vi "Festo Display.vi"() -> ()   [LabVIEW 2011]
uses:
  GlobalVariables.vi
panel:
  in  "Read/Write":bool
  in  "Festo Block 8":bool[][](array[boolean])=[[FALSE, FALSE], [FALSE, FALSE], [FALSE, FALSE], [FALSE, FALSE], [FALSE, FALSE], [FALSE, FALSE], [FALSE, FALSE], [FALSE, FALSE]]
  in  "Festo Block 7":bool[][](array[boolean])=[[FALSE, FALSE], [FALSE, FALSE], [FALSE, FALSE], [FALSE, FALSE], [FALSE, FALSE], [FALSE, FALSE], [FALSE, FALSE], [FALSE, FALSE]]
  in  "Festo Block 6":bool[][](array[boolean])=[[FALSE, FALSE], [FALSE, FALSE], [FALSE, FALSE], [FALSE, FALSE], [FALSE, FALSE], [FALSE, FALSE], [FALSE, FALSE], [FALSE, FALSE]]
  in  "Festo Block 5":bool[][](array[boolean])=[[FALSE, FALSE], [FALSE, FALSE], [FALSE, FALSE], [FALSE, FALSE], [FALSE, FALSE], [FALSE, FALSE], [FALSE, FALSE], [FALSE, FALSE]]
  in  "Festo Block 4":bool[][](array[boolean])=[[FALSE, FALSE], [FALSE, FALSE], [FALSE, FALSE], [FALSE, FALSE], [FALSE, FALSE], [FALSE, FALSE], [FALSE, FALSE], [FALSE, FALSE]]
  in  "Festo Block 3":bool[][](array[boolean])=[[FALSE, FALSE], [FALSE, FALSE], [FALSE, FALSE], [FALSE, FALSE], [FALSE, FALSE], [FALSE, FALSE], [FALSE, FALSE], [FALSE, FALSE]]
  in  "Festo Block 2":bool[][](array[boolean])=[[FALSE, FALSE], [FALSE, FALSE], [FALSE, FALSE], [FALSE, FALSE], [FALSE, FALSE], [FALSE, FALSE], [FALSE, FALSE], [FALSE, FALSE]]
  in  "Festo Block 1":bool[][](array[boolean])=[[FALSE, FALSE], [FALSE, FALSE], [FALSE, FALSE], [FALSE, FALSE], [FALSE, FALSE], [FALSE, FALSE], [FALSE, FALSE], [FALSE, FALSE]]
  in  "Close All Valves":bool
  in  "stop":bool
  # "79\n77\n75\n73\n71\n69\n67\n65"
  # "80\n78\n76\n74\n72\n70\n68\n66"
  # "50\n52\n54\n56\n58\n60\n62\n64"
  # "49\n51\n53\n55\n57\n59\n61\n63"
  # "95\n93\n91\n89\n87\n85\n83\n81"
  # "96\n94\n92\n90\n88\n86\n84\n82"
  # "34\n36\n38\n40\n42\n44\n46\n48"
  # "33\n35\n37\n39\n41\n43\n45\n47"
  # "111\n109\n107\n105\n103\n101\n99\n97"
  # "112\n110\n108\n106\n104\n102\n100\n98"
  # "18\n20\n22\n24\n26\n28\n30\n32"
  # "17\n19\n21\n23\n25\n27\n29\n31"
  # "127\n125\n123\n121\n119\n117\n115\n113"
  # "128\n126\n124\n122\n120\n118\n116\n114"
  # "2\n4\n6\n8\n10\n12\n14\n16"
  # "1\n3\n5\n7\n9\n11\n13\n15"
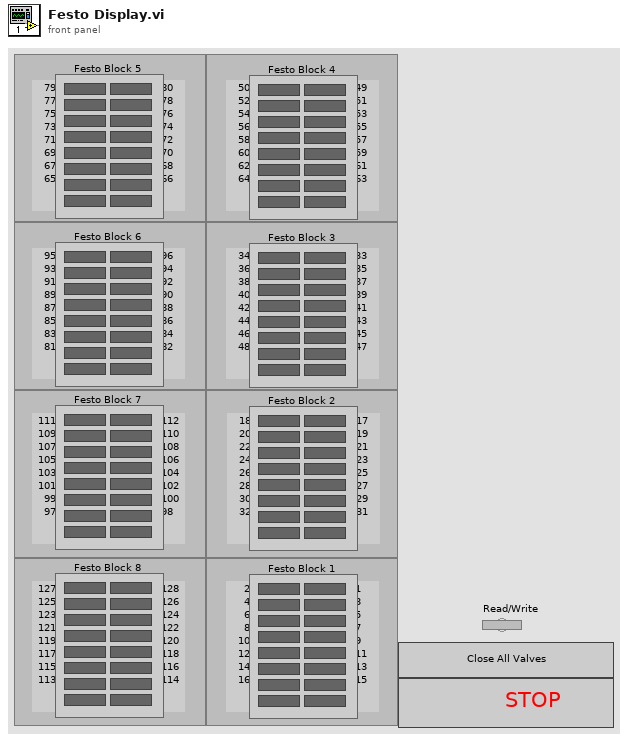
[diagram p1: front panel]
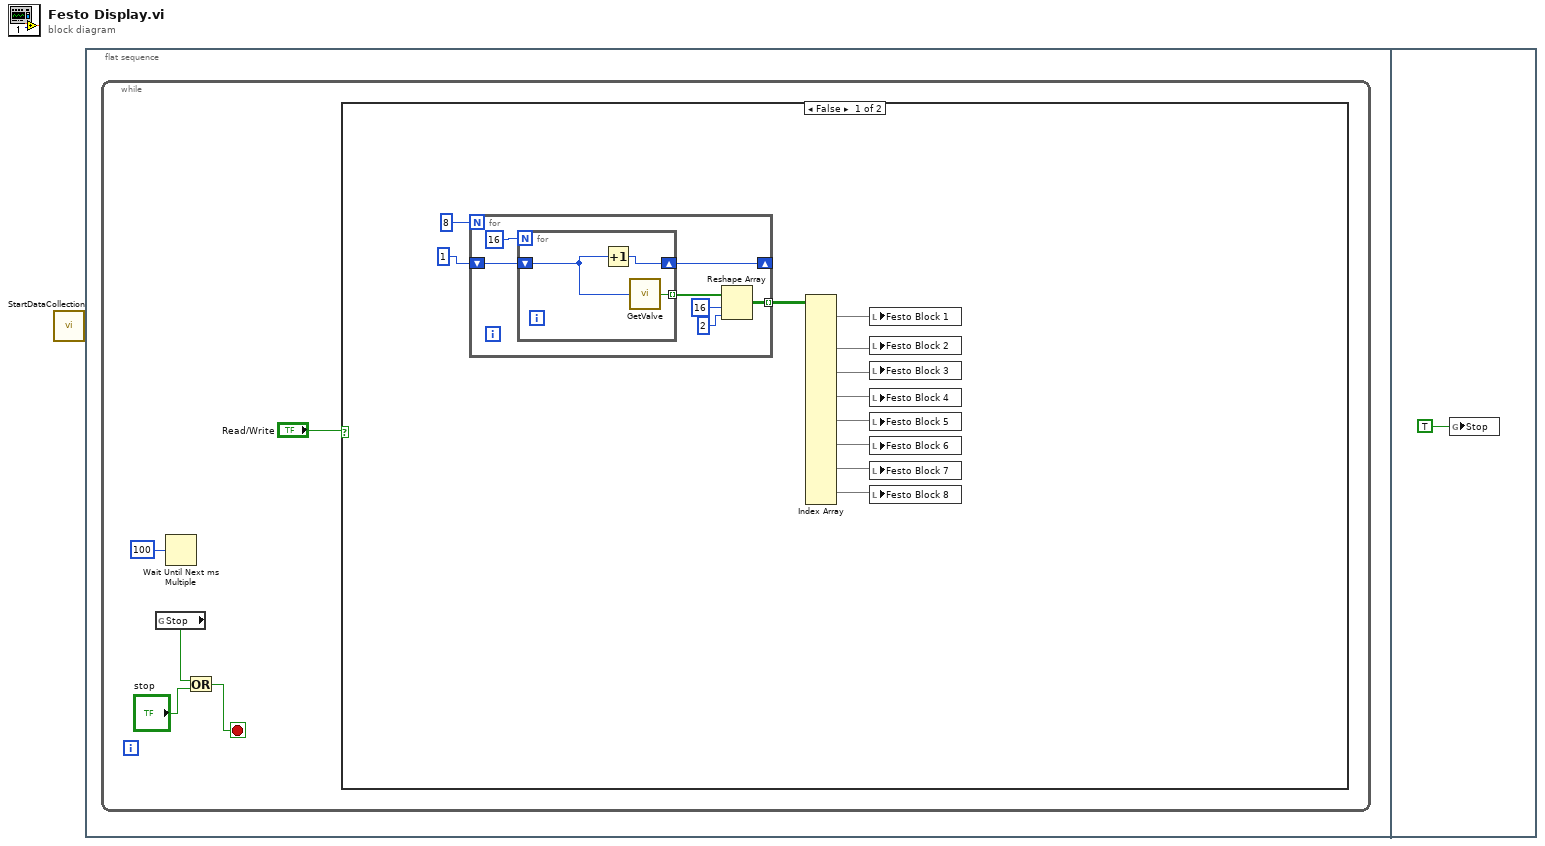
[diagram p0: block diagram]
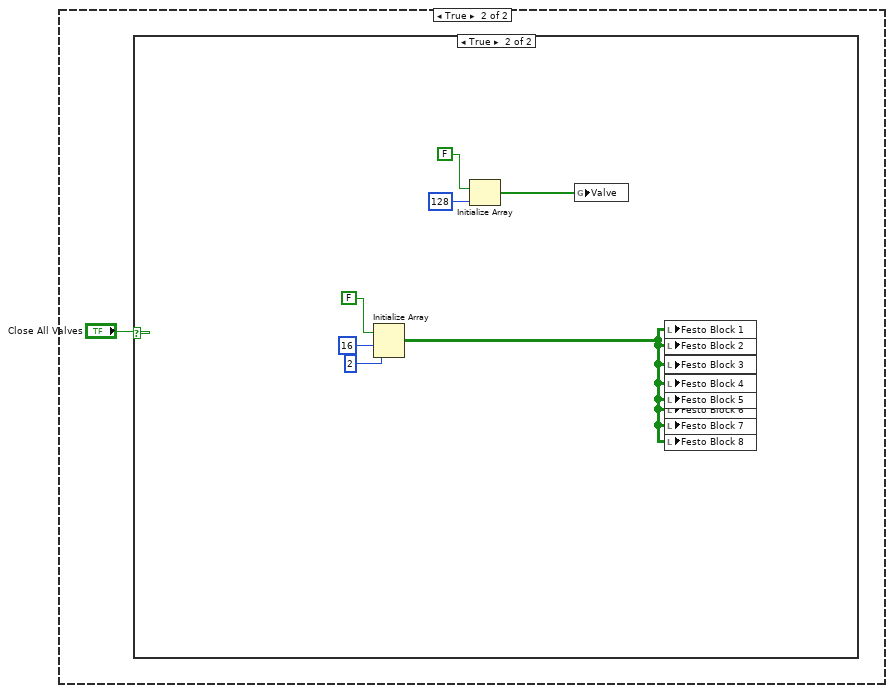
[diagram p2: hidden frame]
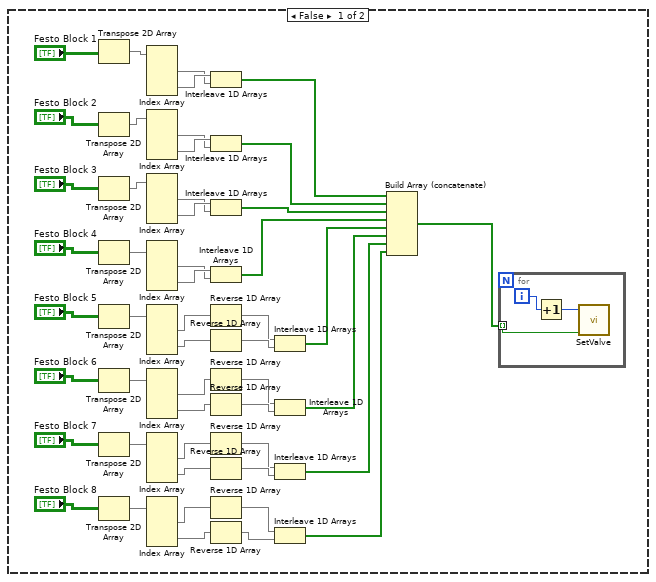
[diagram p3: hidden frame]
diagram:
  n1 = call "StartDataCollection.vi"() -> ()  [unwired: 12 in]
  n2 = flat-sequence {
    frame #0 {
      n3 = while {
        stop <- w2 stop-if-true
        n4 = global read "GlobalVariables.vi" "Stop"() -> (w3:bool)
        n5 = Wait Until Next ms Multiple(millisecond multiple=100) -> ()  [unwired: 1 out]
        n6 = Or(x=w3, y="stop") -> (x .or. y?=w2:bool)
        n7 = case shown="False" "Read/Write" {
          frame False {
            n8 = for {
              N: 8 -> [_]
              tunnel: [w19] -> w15 mode=indexing
              shift-right: [w17] -> _
              shift-left: 1 -> [w18]
              n9 = for {
                N: 16 -> [_]
                tunnel: [w26] -> w22 mode=indexing
                shift-right: [w24] -> w17
                shift-left: w18 -> [w25]
                n10 = Increment(x=w25) -> (x+1=w24:i32)
                n11 = call "GetValve.vi"("Numeric"=w25) -> ("Boolean"=w26:bool)
              }
              n12 = Reshape Array(w22, 16 ("dimension size"), 2 ("dimension size")) -> (w19:bool[][])
            }
            n13 = Index Array(array=w15) -> (element #1=w14:bool[][], element #2=w13:bool[][], element #3=w12:bool[][], element #4=w11:bool[][], element #5=w10:bool[][], element #6=w9:bool[][], element #7=w8:bool[][], element #8=w7:bool[][])  [unwired: 24 in]
            n14 = local write "Festo Block 1"(w14) -> ()
            n15 = local write "Festo Block 2"(w13) -> ()
            n16 = local write "Festo Block 3"(w12) -> ()
            n17 = local write "Festo Block 4"(w11) -> ()
            n18 = local write "Festo Block 5"(w10) -> ()
            n19 = local write "Festo Block 6"(w9) -> ()
            n20 = local write "Festo Block 7"(w8) -> ()
            n21 = local write "Festo Block 8"(w7) -> ()
          }
          frame True {
            n22 = case shown="True" "Close All Valves" {
              frame False {
                n23 = Transpose 2D Array(2D array="Festo Block 1") -> (transposed array=w43:bool[][])
                n24 = Transpose 2D Array(2D array="Festo Block 2") -> (transposed array=w35:bool[][])
                n25 = Transpose 2D Array(2D array="Festo Block 3") -> (transposed array=w34:bool[][])
                n26 = Transpose 2D Array(2D array="Festo Block 4") -> (transposed array=w33:bool[][])
                n27 = Transpose 2D Array(2D array="Festo Block 5") -> (transposed array=w32:bool[][])
                n28 = Transpose 2D Array(2D array="Festo Block 6") -> (transposed array=w31:bool[][])
                n29 = Transpose 2D Array(2D array="Festo Block 7") -> (transposed array=w30:bool[][])
                n30 = Transpose 2D Array(2D array="Festo Block 8") -> (transposed array=w29:bool[][])
                n31 = Index Array(array=w43) -> (element #1=w75:bool[], element #2=w76:bool[])  [unwired: 4 in]
                n32 = Index Array(array=w35) -> (element #1=w73:bool[], element #2=w74:bool[])  [unwired: 4 in]
                n33 = Index Array(array=w34) -> (element #1=w71:bool[], element #2=w72:bool[])  [unwired: 4 in]
                n34 = Index Array(array=w33) -> (element #1=w69:bool[], element #2=w70:bool[])  [unwired: 4 in]
                n35 = Index Array(array=w32) -> (element #1=w68:bool[], element #2=w67:bool[])  [unwired: 4 in]
                n36 = Index Array(array=w31) -> (element #1=w66:bool[], element #2=w65:bool[])  [unwired: 4 in]
                n37 = Index Array(array=w30) -> (element #1=w61:bool[], element #2=w62:bool[])  [unwired: 4 in]
                n38 = Index Array(array=w29) -> (element #1=w64:bool[], element #2=w63:bool[])  [unwired: 4 in]
                n39 = Interleave 1D Arrays(w76, w75) -> (w52:bool[])
                n40 = Interleave 1D Arrays(w74, w73) -> (w51:bool[])
                n41 = Interleave 1D Arrays(w72, w71) -> (w50:bool[])
                n42 = Interleave 1D Arrays(w70, w69) -> (w49:bool[])
                n43 = Reverse 1D Array(array=w68) -> (reversed array=w53:bool[])
                n44 = Reverse 1D Array(array=w67) -> (reversed array=w54:bool[])
                n45 = Reverse 1D Array(array=w66) -> (reversed array=w55:bool[])
                n46 = Reverse 1D Array(array=w65) -> (reversed array=w56:bool[])
                n47 = Reverse 1D Array(array=w61) -> (reversed array=w57:bool[])
                n48 = Reverse 1D Array(array=w62) -> (reversed array=w58:bool[])
                n49 = Reverse 1D Array(array=w64) -> (reversed array=w59:bool[])
                n50 = Reverse 1D Array(array=w63) -> (reversed array=w60:bool[])
                n51 = Interleave 1D Arrays(w53, w54) -> (w48:bool[])
                n52 = Interleave 1D Arrays(w55, w56) -> (w47:bool[])
                n53 = Interleave 1D Arrays(w57, w58) -> (w46:bool[])
                n54 = Interleave 1D Arrays(w59, w60) -> (w45:bool[])
                n55 = Build Array (concatenate)(w52, w51, w50, w49, w48, w47, w46, w45) -> (w28:bool[])
                n56 = for {
                  tunnel: w28 -> [w79] mode=indexing
                  i -> [w78]
                  n57 = Increment(x=w78) -> (x+1=w77:i32)
                  n58 = call "SetValve.vi"("Open/Close"=w79, "Valve"=w77) -> ()  [unwired: 10 in]
                }
              }
              frame True {
                n59 = Initialize Array(FALSE, 16 ("dimension size"), 2 ("dimension size")) -> (w80:bool[][])
                n60 = Initialize Array(FALSE, 128 ("dimension size")) -> (w84:bool[])
                n61 = global write "GlobalVariables.vi" "Valve"(w84) -> ()
                n62 = local write "Festo Block 1"(w80) -> ()
                n63 = local write "Festo Block 2"(w80) -> ()
                n64 = local write "Festo Block 3"(w80) -> ()
                n65 = local write "Festo Block 4"(w80) -> ()
                n66 = local write "Festo Block 5"(w80) -> ()
                n67 = local write "Festo Block 6"(w80) -> ()
                n68 = local write "Festo Block 7"(w80) -> ()
                n69 = local write "Festo Block 8"(w80) -> ()
              }
            }
          }
        }
      }
    }
    frame #1 {
      n70 = global write "GlobalVariables.vi" "Stop"(TRUE ("Stop")) -> ()
    }
  }
